vi "Write Module Error Configurations.vi"(7 "Module ID":string, 8 "error in":errorcluster, 10 "Module Error Configuration":T1, 11 "Standard Engine Repo Data in":refnum<class "Standard Engine Configuration.lvclass">) -> (0 "error out":errorcluster, 3 "Standard Engine Repo Data out":refnum<class "Standard Engine Configuration.lvclass">)   [LabVIEW 2013, in "Standard Engine Configuration.lvclass"]
uses:
  Standard Engine Configuration.lvclass
  Module Error Configuration.ctl
  Error Actions By Category.ctl
  <vilib>/NI/Tag Bus Module Framework/runtime/error classification.ctl
  Error Actions.ctl
  Standard Engine Configuration.lvclass/Standard Engine Configuration.ctl
  <vilib>/NI/Tag Bus Module Framework/runtime/TBM module execution interface.lvclass
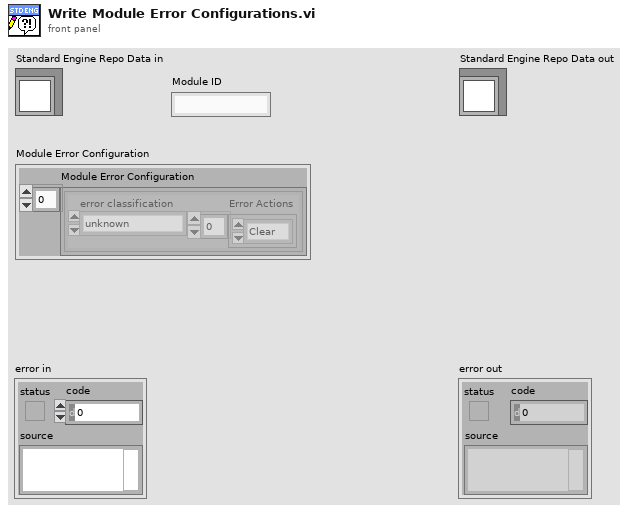
[diagram p1: front panel]
types:
  T1 = typedef "Standard Engine Configuration.lvclass/Module Error Configuration.ctl" = cluster{"Module Error Configuration":T2[]}
  T2 = typedef "Standard Engine Configuration.lvclass/Error Actions By Category.ctl" = cluster{"error classification":T3, "Error Actions":T4[]}
  T3 = typedef "TBM module execution interface.lvclass/error classification.ctl" = enum16{"unknown", "none", "trivial", "recoverable", "critical"}
  T4 = typedef "Standard Engine Configuration.lvclass/Error Actions.ctl" = enum16{"Clear", "Notify", "Stop Component", "Stop Engine", "Safe State", "Attempt Recovery"}
  T5 = typedef "Standard Engine Configuration.lvclass/Module Specific Configuration.ctl" = cluster{"Module ID":string, "Module Decimation":T6, "Module Error Configuration":T1, "execution order priority":i32, "async?":bool, "error tag":string}
  T6 = typedef "Standard Engine Configuration.lvclass/Module Decimation.ctl" = cluster{"Decimation":u16, "Offset":u16}
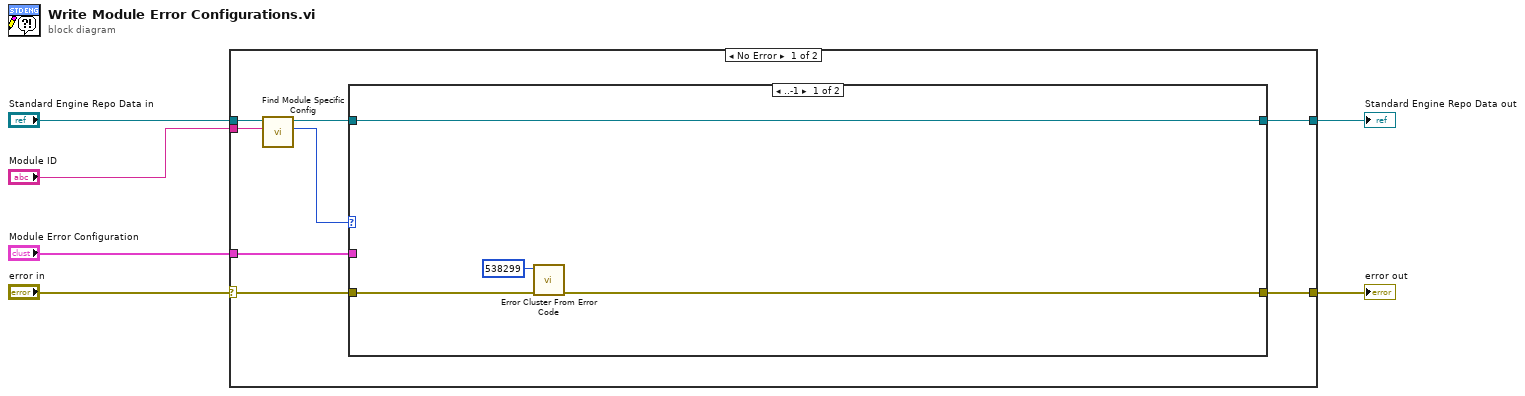
[diagram p0: block diagram]
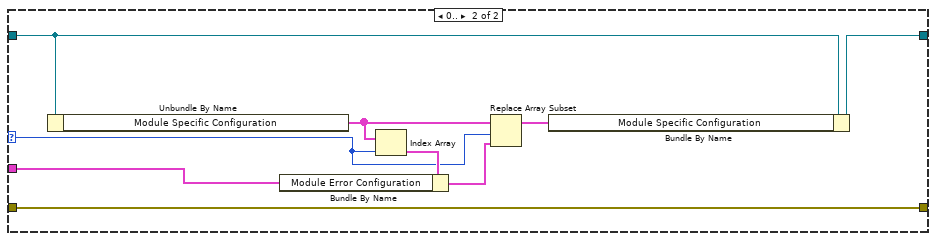
[diagram p2: hidden frame]
diagram:
  n1 = case shown="No Error" "error in" {
    selector: "error in" -> [w10 w29]
    tunnel: "Standard Engine Repo Data in" -> [w14 w28]
    tunnel: "Module ID" -> [w13 _]
    tunnel: [w8 w28] -> w2
    tunnel: [w9 w29] -> w1
    tunnel: "Module Error Configuration" -> [w7 _]
    frame No Error {
      n2 = call "Find Module Specific Config.vi"("Module ID"=w13, "Standard Engine Repo Data in"=w14) -> ("Index"=w11:i32, "Standard Engine Repo Data out"=w12:refnum<class "Standard Engine Configuration.lvclass">)  [unwired: 8 in]
      n3 = case shown="..-1" w11 {
        selector: w11 -> [_ w24]
        tunnel: w12 -> [w17 w21]
        tunnel: w10 -> [w18 w27]
        tunnel: [w16 w27] -> w9
        tunnel: [w17 w19] -> w8
        tunnel: w7 -> [_ w25]
        frame ..-1 {
          n4 = call <vilib>:"Error Cluster From Error Code.vi"("error in (no error)"=w18, "error code (0)"=538299) -> ("error out"=w16:errorcluster)  [unwired: 7 in]
        }
        frame 0.. {
          n5 = Unbundle By Name(w21) -> ("Module Specific Configuration"=w23:T5[])
          n6 = Index Array(array=w23, index=w24) -> (element=w26:T5)
          n7 = Bundle By Name(cluster=w26, "Module Error Configuration"=w25) -> (w22:T5)
          n8 = Replace Array Subset(array=w23, new element=w22, index=w24) -> (w20:T5[])
          n9 = Bundle By Name(cluster=w21, "Module Specific Configuration"=w20) -> (w19:refnum<class "Standard Engine Configuration.lvclass">)
        }
      }
    }
    frame Error {
    }
  }
  "error out" <- w1
  "Standard Engine Repo Data out" <- w2
